vi "Microchip 93LC56BT Write.vi"() -> ()   [LabVIEW 2015]
doc: "This example shows a more generalized way to use the SPI advanced API to write data. It allows the user to change the following parameters: page size, write delay, the endianness of the address bytes, and the number of bytes in an address.\n\nThe parameters will have the following effects:\n\nTarget Page Size (bytes): This places an additional constraint on the amount of bytes written. The smaller value will be used, and that number of bytes written.\nWrite Delay Between Pages (ms): This will force a mandatory delay after writing bytes to a device.\nData Address Width: This will allow the user to specify the EEPROM Data Address as either 1 or 2 bytes.\nData Address Endianness: This control will change the ordering of the bytes in the EEPROM Data Address, note that this only has an effect if there are 2 bytes in the address.\n\nFor connection information see the NI-845x Hardware and Software manual and the manual for your specific SPI device."
uses:
  <vilib>/ni845x/ni845x.llb/ni845xControl.ctl
  <vilib>/ni845x/ni845x.llb/ni845xSpiScriptControl.ctl
  <vilib>/ni845x/ni845x.llb/NI-845x SPI Script Ms Delay.vi
  <vilib>/ni845x/ni845x.llb/NI-845x SPI Close Script Reference.vi
  <resource>/objmgr/NI845x.rc
panel:
  in  "EWEN":u8=19 format="%08b"
  in  "READ":u8=6 format="%08b"
  in  "WRITE":u8=5 format="%08b"
  in  "Read Device":bool
  in  "Program Device":bool
  out "Read Data":u16[](array[numeric]) format="%x"
  in  "EWDS":u8=16 format="%08b"
  in  "CS Idle":enum16{"Low (Assert High)", "High (Assert Low)"}(ring)
  in  "clock phase":i32(ring) items=["0 (First Edge)", "1 (Second Edge)"]
  in  "clock polarity":i32(ring) items=["0 (Idle Low)", "1 (Idle High)"]
  in  "SPI Script Reference":T1
  in  "QUIT":bool
  in  "Bit Pattern":T2(ring)
  in  "I/O Voltage Level":i32(ring)=33 items=["3.3V"=33, "2.5V"=25, "1.8V"=18, "1.5V"=15, "1.2V"=12]
  in  "Data Address Endianness":bool=TRUE
  in  "Chip Select":u32
  in  "Data Address Width":enum16{"1 Byte", "2 Byte"}(ring)
  in  "Page Write Delay (ms)":u32=3
  in  "Target Page Size (bytes)":u32=2
  in  "NI8451 Device ID":T3="NI-8451"
  in  "EEPROM Data Address":u8 format="%.0x"
  in  "Number of Bytes (Read/Write)":u32=2
  in  "Clock Rate (kHz)":u16=2000
  out "Data Bytes Written":u8[](array[numeric]) format="%x"
  # "SPI Slave Configuration"
  # "SPI Data"
  # "NI-USB-8451 Device Configuration"
  # "Big Endian"
  # "Little Endian"
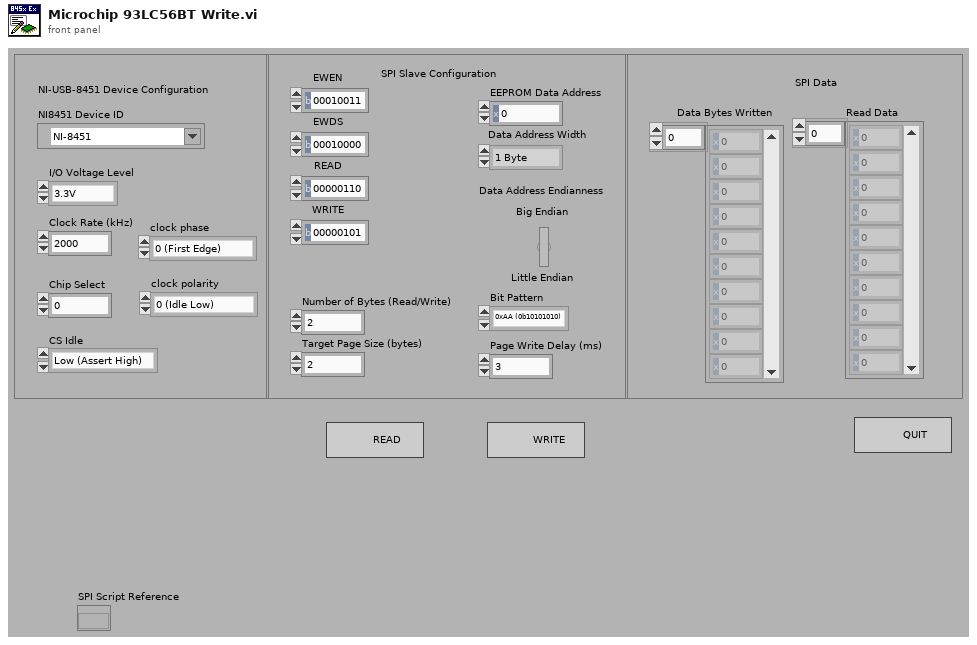
[diagram p1: front panel]
types:
  T1 = typedef "ni845xSpiScriptControl.ctl" = refnum<k20>
  T2 = enum16{"0xAA (0b10101010)", "0x55 (0b01010101)", "All ONES", "All ZEROES"}
  T3 = typedef "ni845xControl.ctl" = refnum<k21>
  T4 = enum32{"Invalid", "Standard", "Closed", "Hidden", "Minimized", "Maximized"}
  T5 = enum32{"invalid app kind", "Development System", "Run Time System", "Student Edition", "Embedded LabVIEW", "Evaluation", "Custom"}
  T6 = cluster{"SPI Script Reference":T1, "Core":cluster{"Current VI Reference":refnum<vi>, "Close Panel on Exit?":bool}, "NI8451 Device ID":T3, "I/O Voltage Level":i32, "Chip Select":u32, "Clock Rate (kHz)":u16, "clock polarity":i32, "clock phase":i32, "EEPROM Data Address":u8, "Number of Bytes (Read/Write)":u32, "Target Page Size (bytes)":u32, "Page Write Delay (ms)":u32, "CS Idle":enum16{"Low (Assert High)", "High (Assert Low)"}, "Data Address Width":enum16{"1 Byte", "2 Byte"}, "script read index":u32, "READ":u8, "WRITE":u8, "EWEN":u8, "EWDS":u8, "Data Address Endianness":bool}
  T7 = cluster{"Current VI Reference":refnum<vi>, "Close Panel on Exit?":bool}
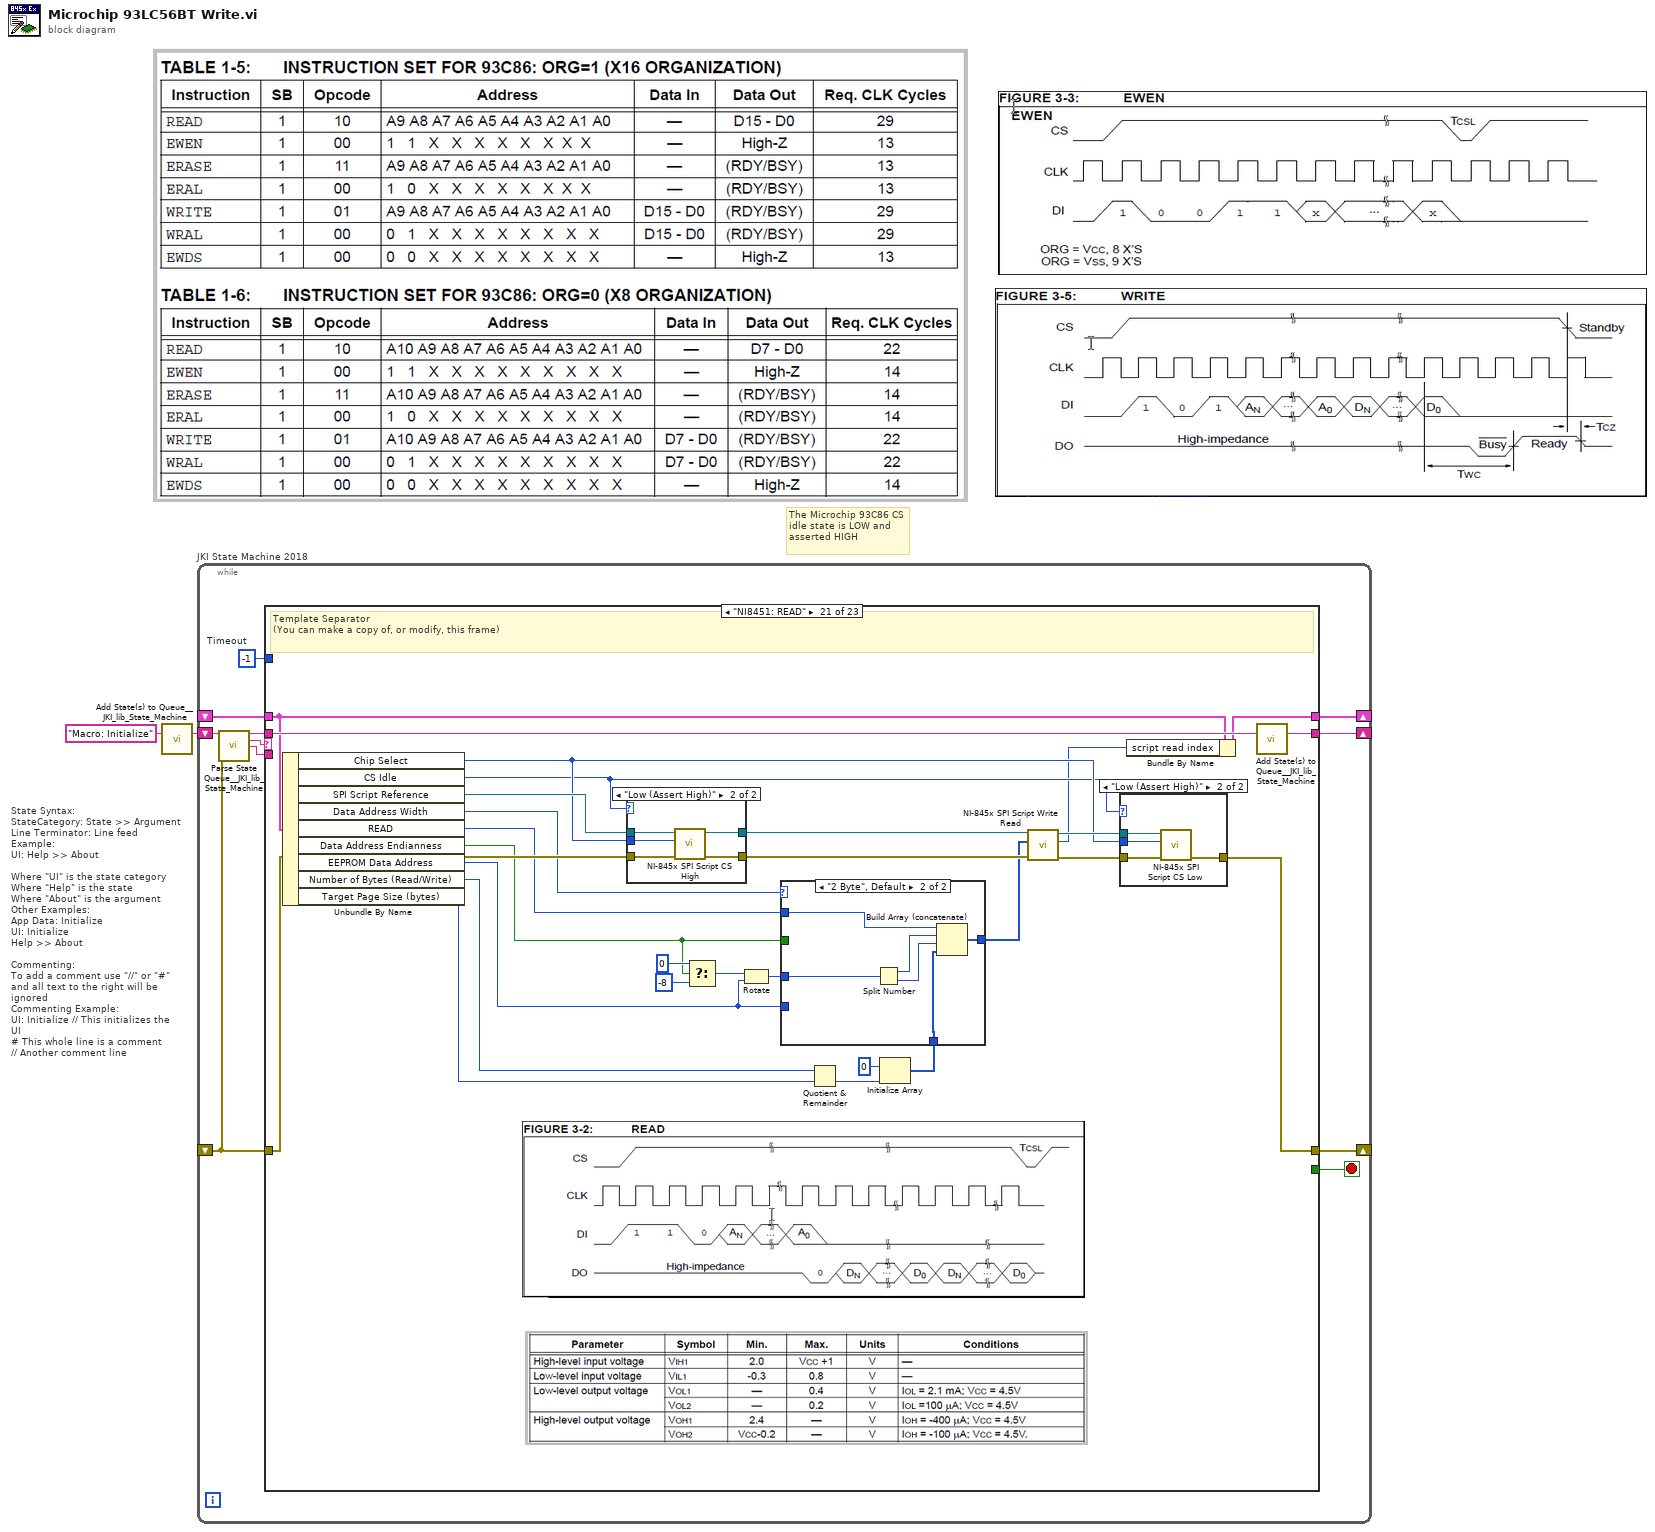
[diagram p0: block diagram]
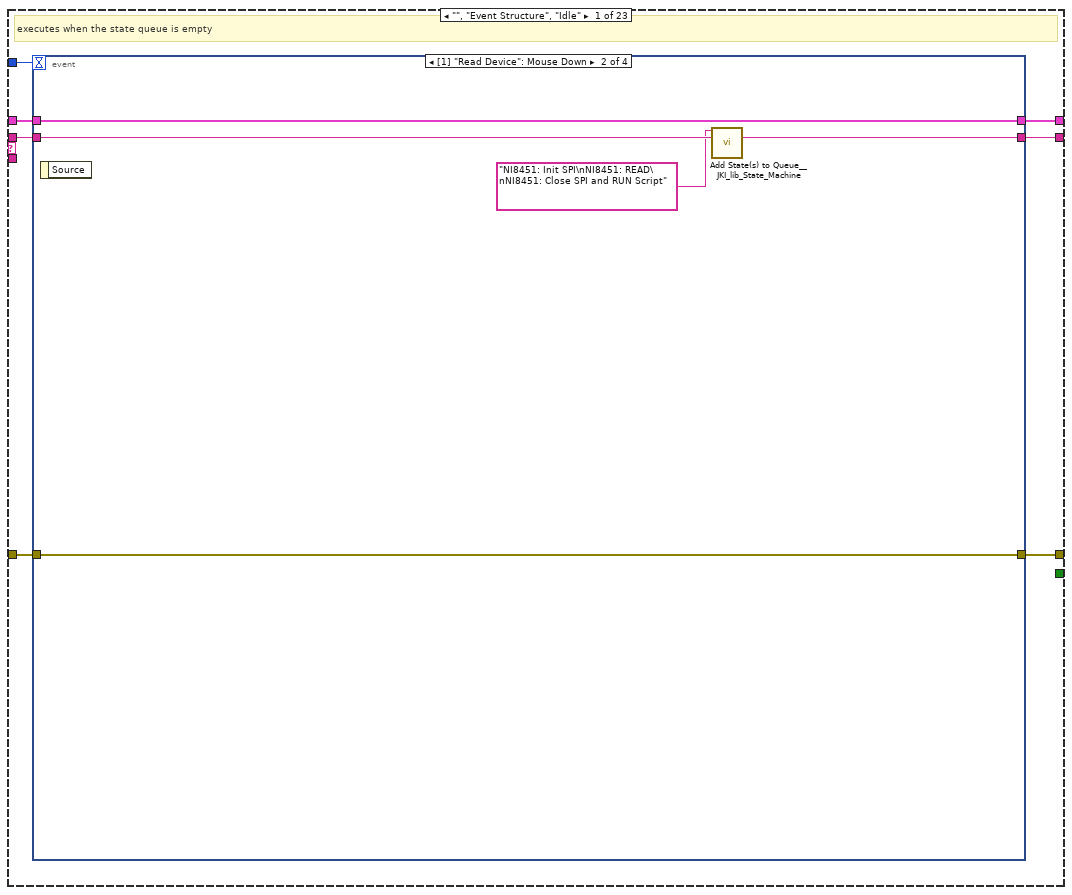
[diagram p2: hidden frame]
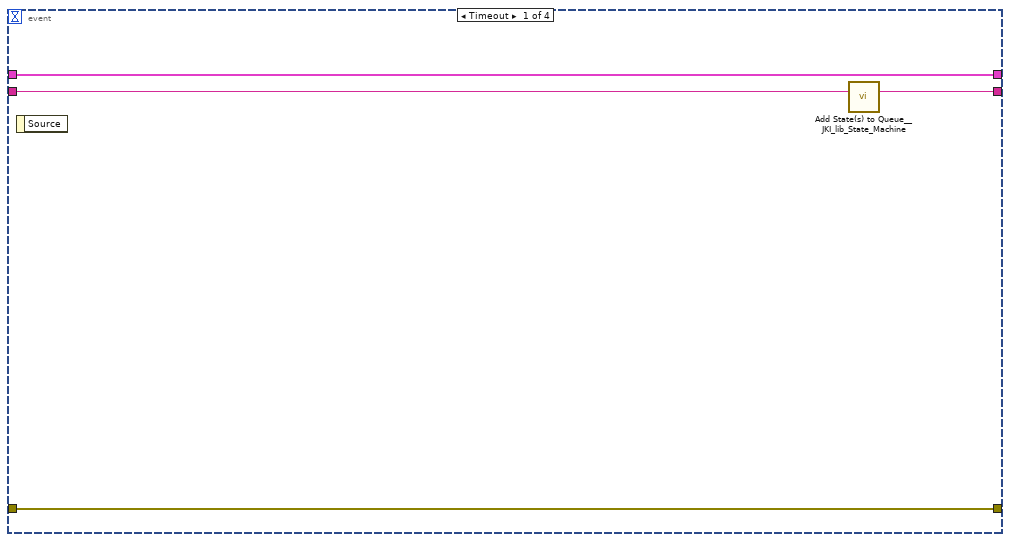
[diagram p3: hidden frame]
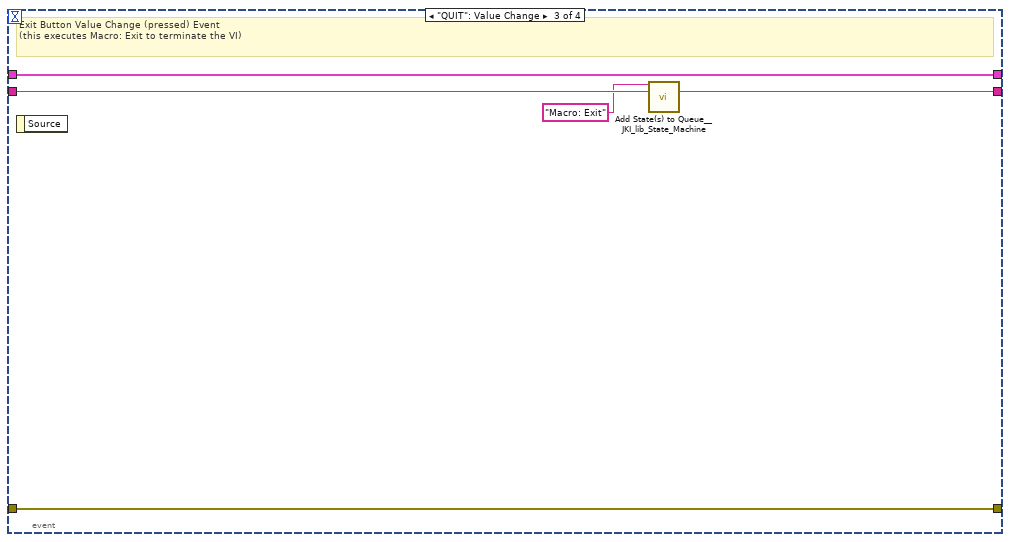
[diagram p4: hidden frame]
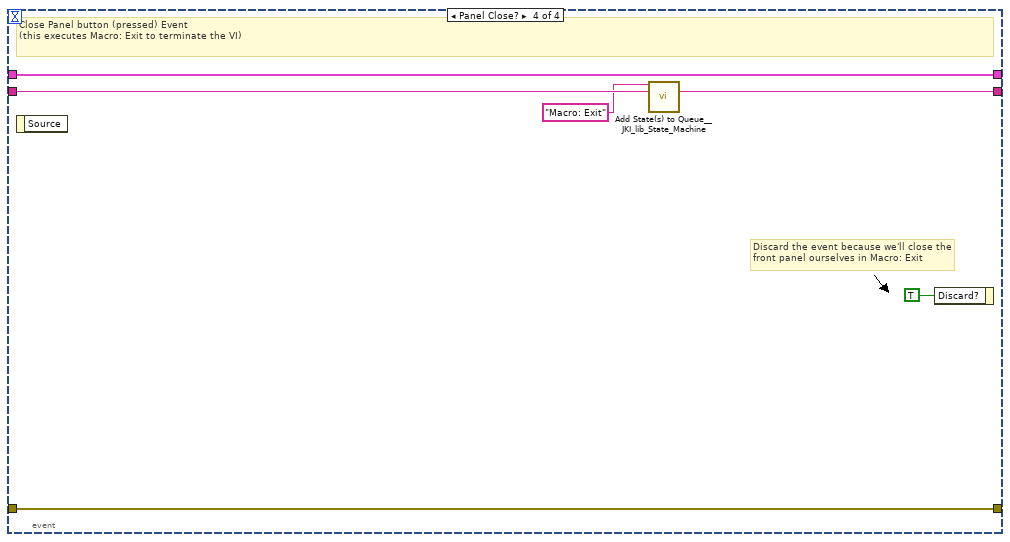
[diagram p5: hidden frame]
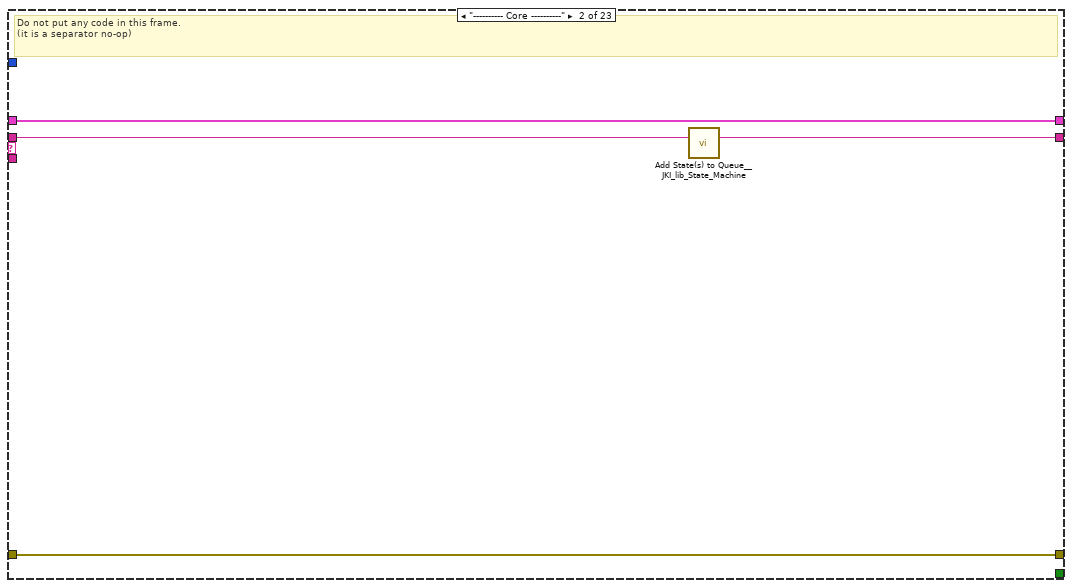
[diagram p6: hidden frame]
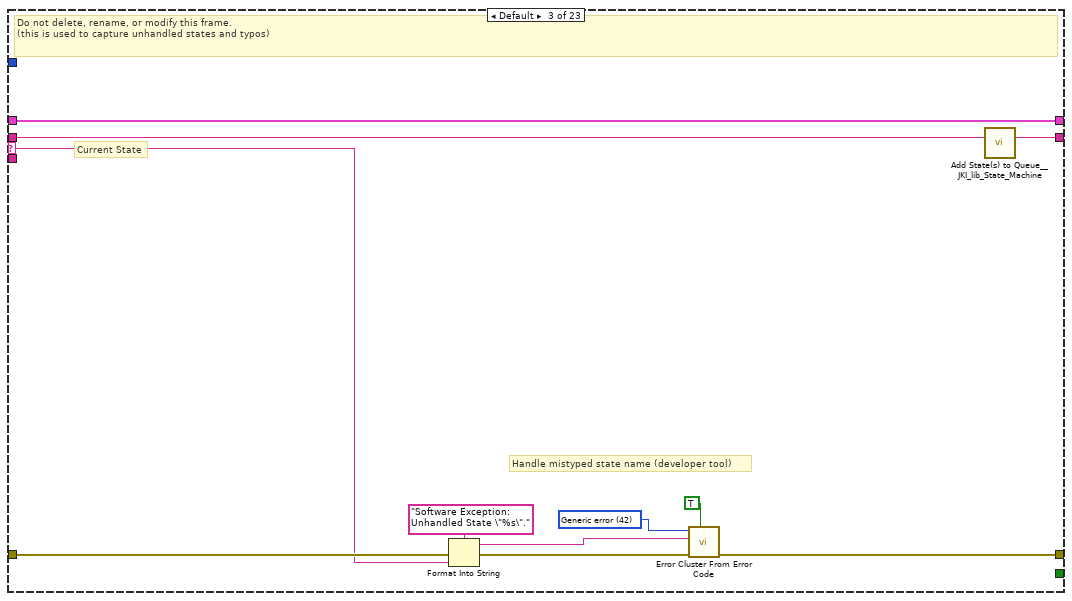
[diagram p7: hidden frame]
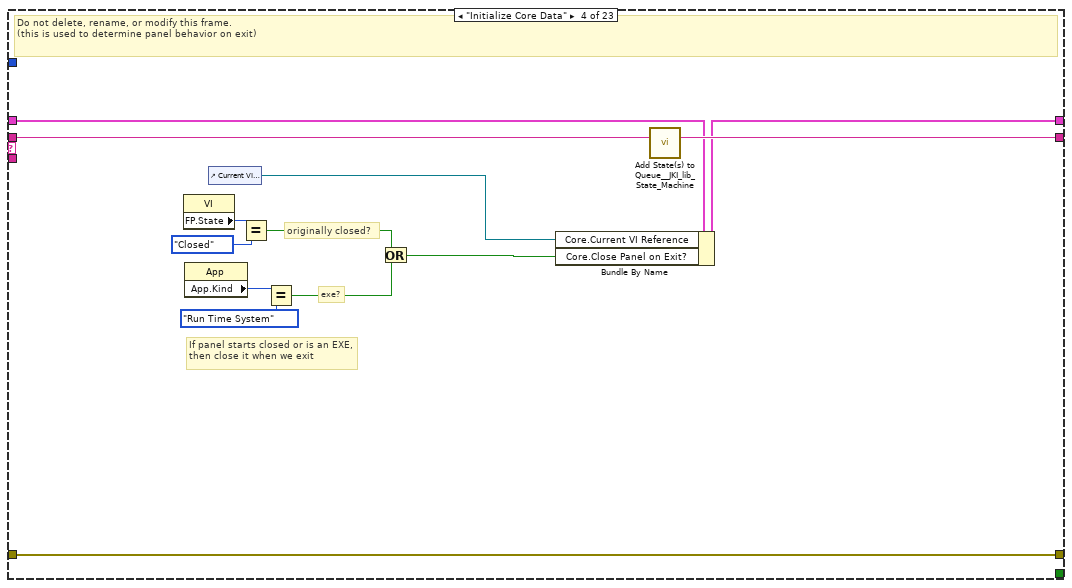
[diagram p8: hidden frame]
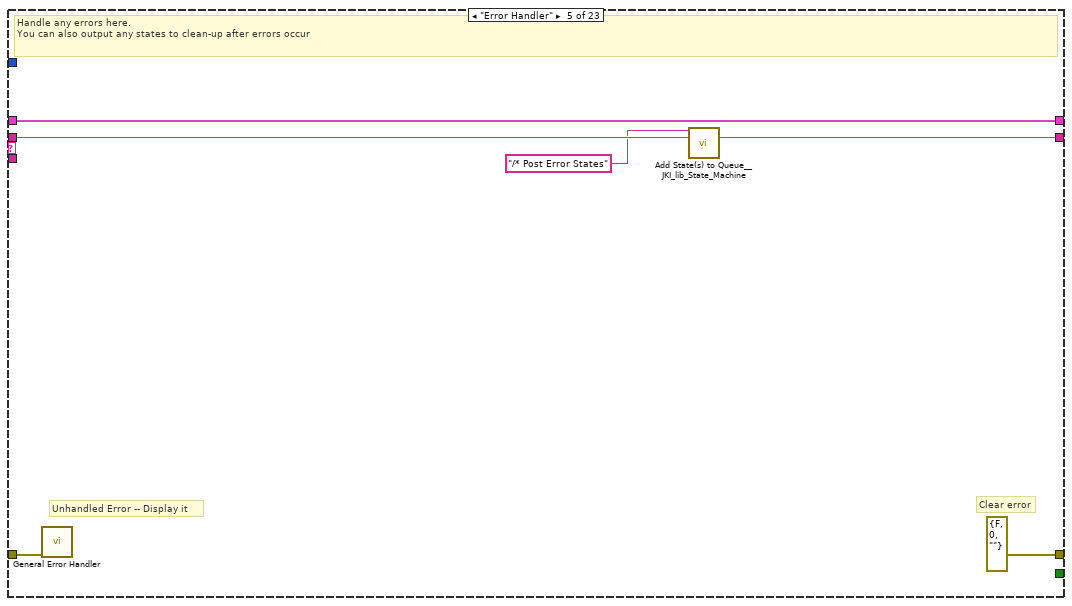
[diagram p9: hidden frame]
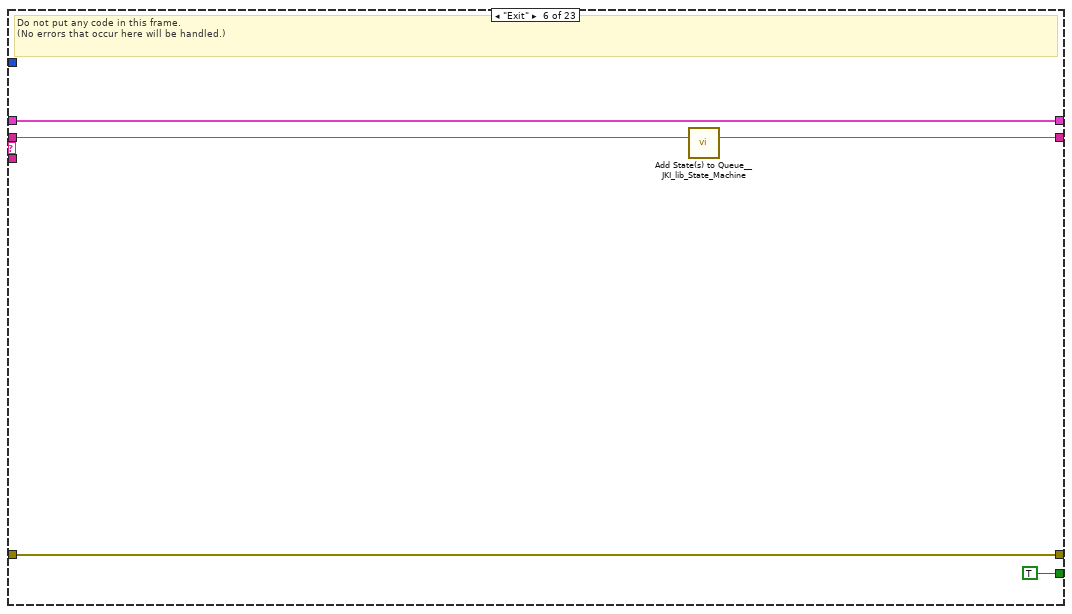
[diagram p10: hidden frame]
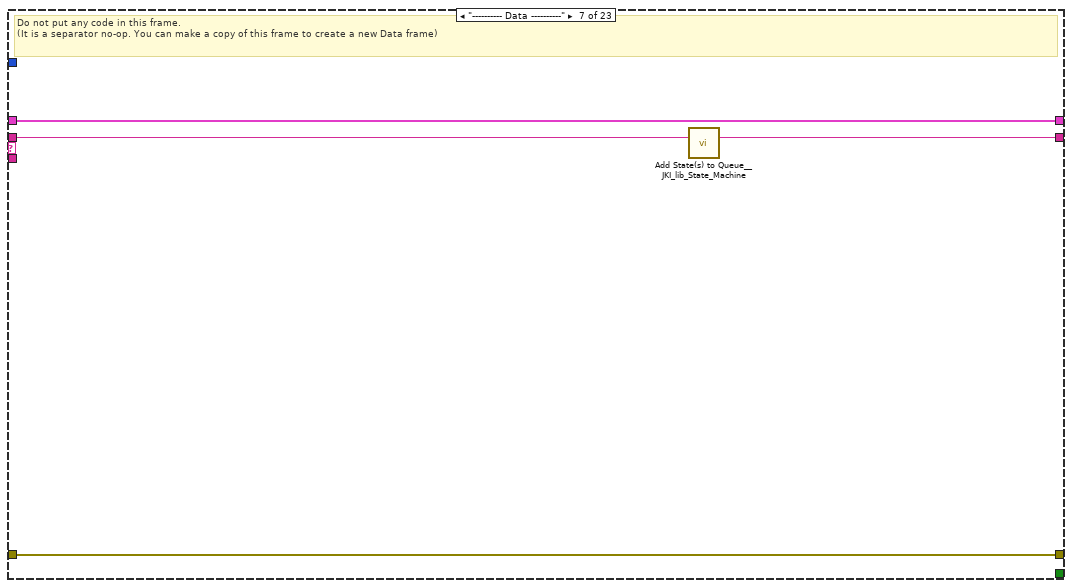
[diagram p11: hidden frame]
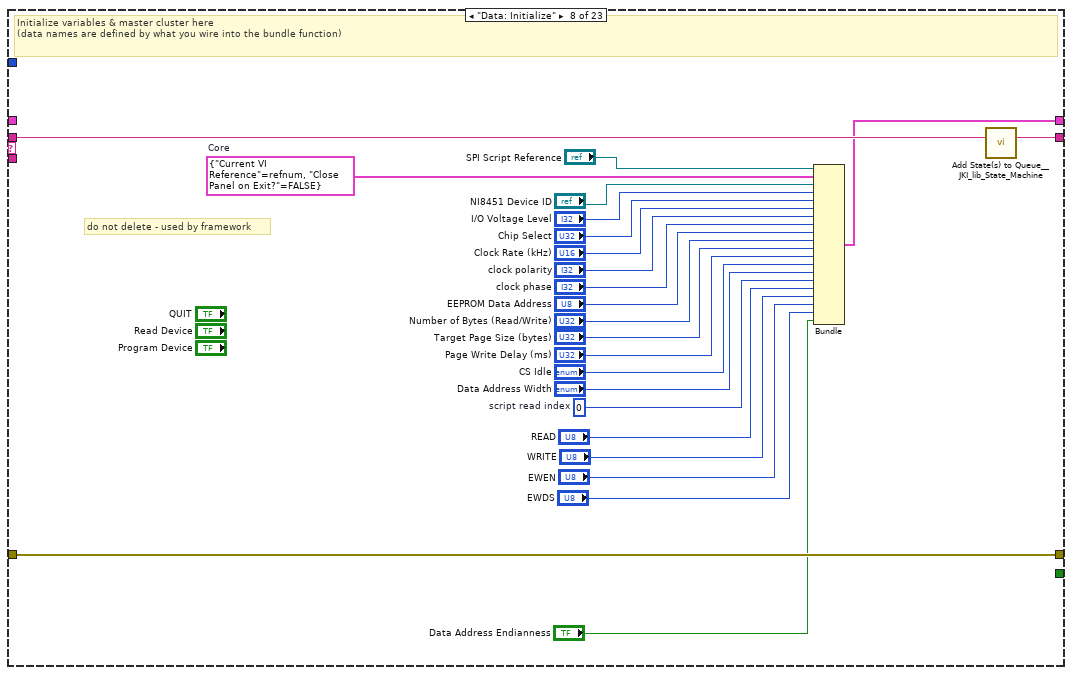
[diagram p12: hidden frame]
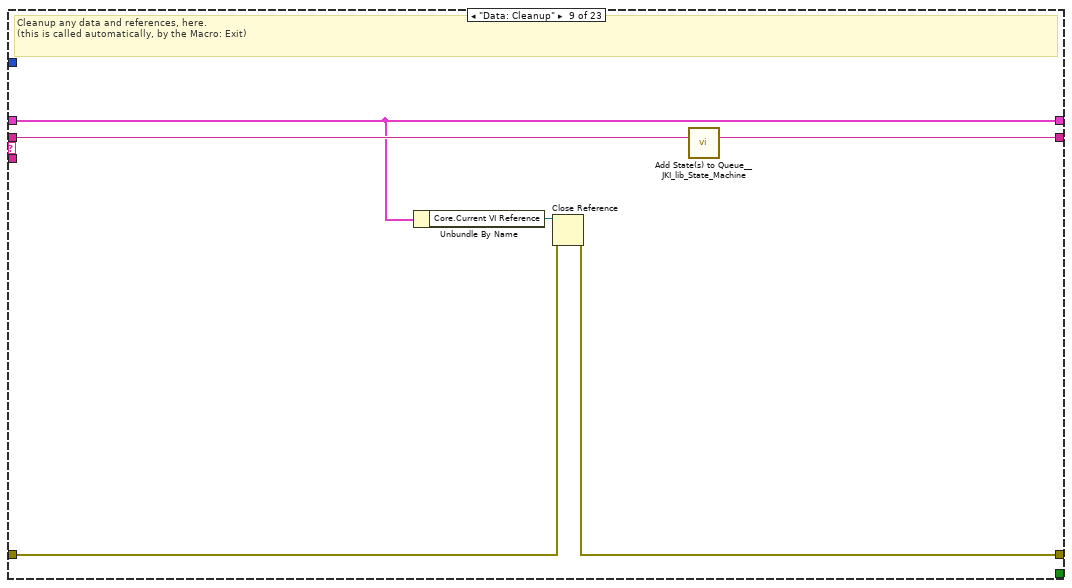
[diagram p13: hidden frame]
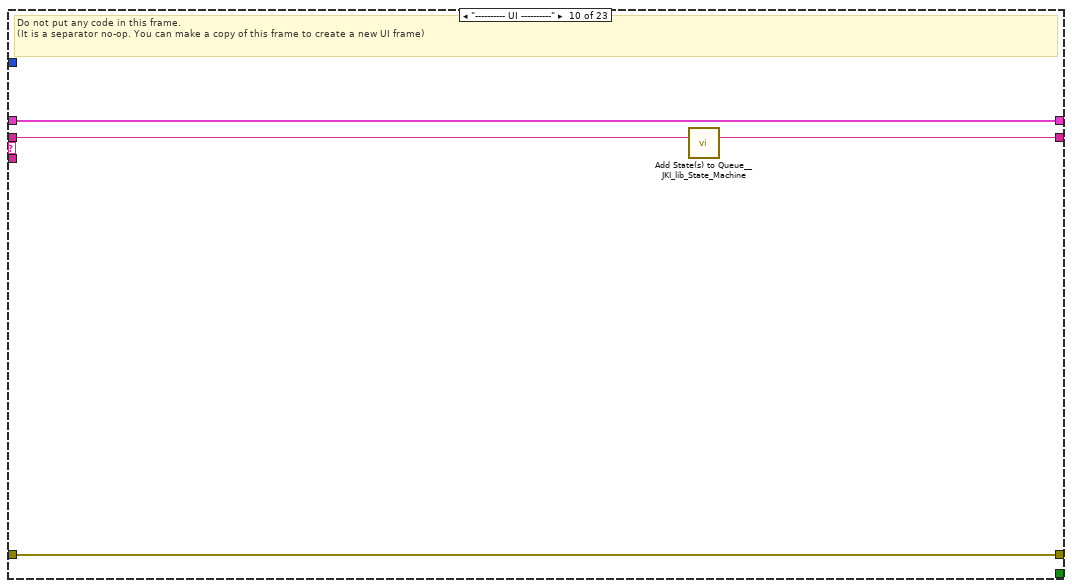
[diagram p14: hidden frame]
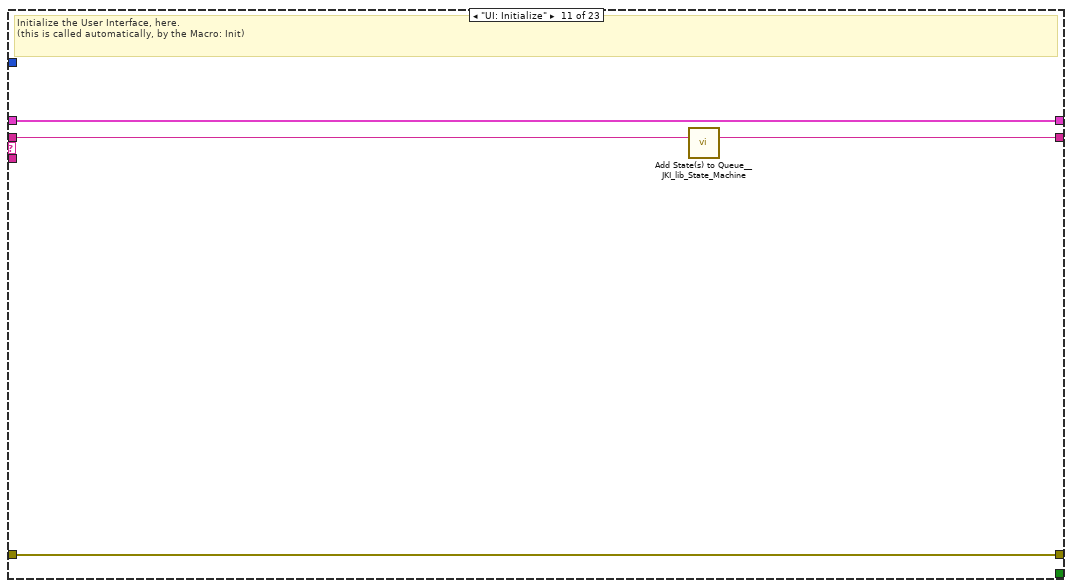
[diagram p15: hidden frame]
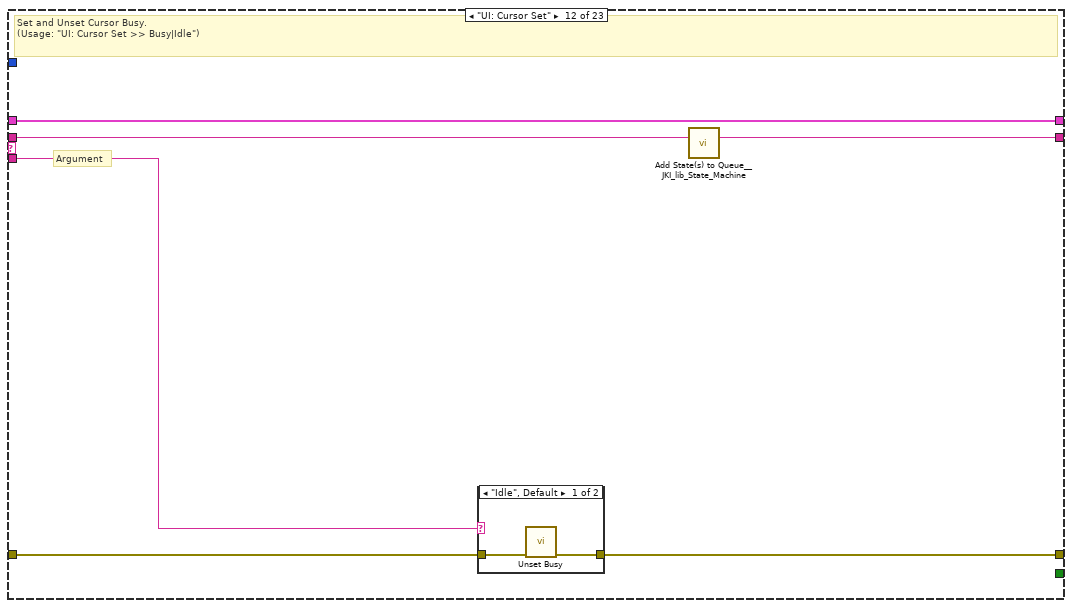
[diagram p16: hidden frame]
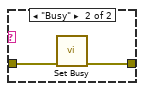
[diagram p17: hidden frame]
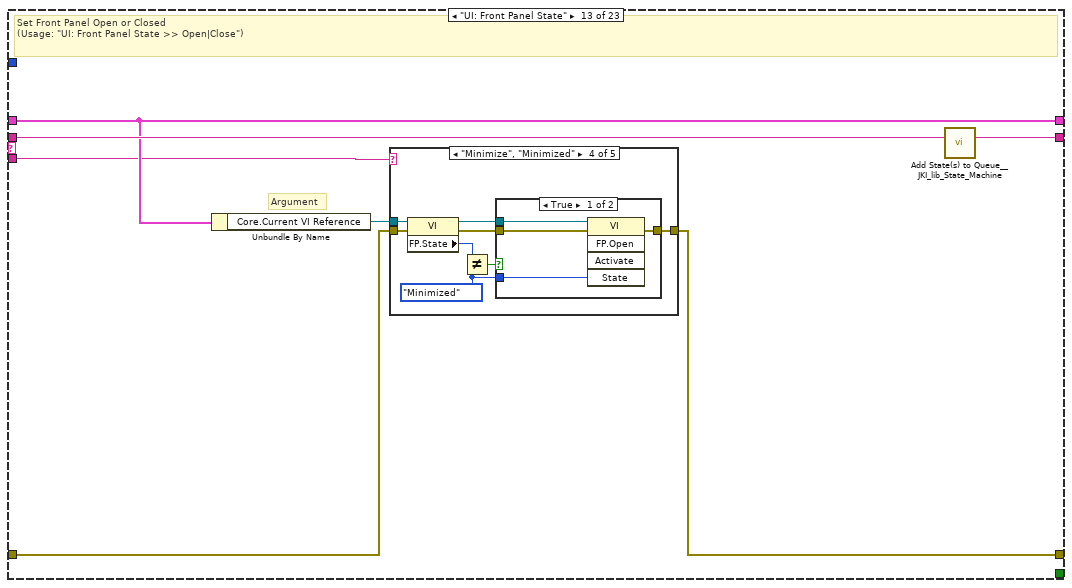
[diagram p18: hidden frame]
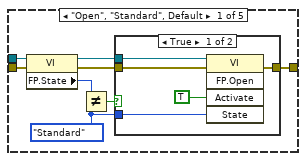
[diagram p19: hidden frame]
diagram:
  # "The Microchip 93C86 CS idle state is LOW and asserted HIGH"
  # "State Syntax:\nStateCategory: State >> Argument\nLine Terminator: Line feed\nExample:\nUI: Help >> About\n\nWhere \"UI\" is the state category\nWhere \"Help\" is the state\nWhere \"About\" is the argument\nOther Examples:\nApp Data: Initialize\nUI: Initialize\nHelp >> About\n\nCommenting:\nTo add a comment use \"//\" or \"#\" and all text to the right will be ignored\nCommenting Example:\nUI: Initialize // This initializes the UI\n# This whole line is a comment\n// Another comment line"
  n1 = call <vilib>:"Add State(s) to Queue__JKI_lib_State_Machine.vi"("State(s) in (\"\")"="Macro: Initialize") -> ("States Out"=w2:string)  [unwired: 14 in]
  n2 = while "JKI State Machine 2018" {
    shift-right: [w6] -> _
    shift-left: _ -> [w5]
    shift-right: [w9] -> _
    shift-left: _ -> [w3]
    shift-right: [w8] -> _
    shift-left: w2 -> [w10]
    stop <- w7 stop-if-true
    w4 = -1  # Timeout
    n3 = call <vilib>:"Parse State Queue__JKI_lib_State_Machine.vi"("State Queue"=w10, "Error In (no error)"=w3) -> ("Remaining States"=w12:string, "Current State"=w13:string, "Arguments"=w11:string)  [unwired: 11 in]
    n4 = case shown="\"NI8451: READ\"" w13 {
      selector: w13 -> [_ _ w45 _ _ _ _ _ _ _ _ _ _ _ _ _ _ _ _ _ _ _ _]
      tunnel: w12 -> [w20 w44 w49 w68 w74 w79 w83 w107 w113 w117 w121 w127 w138 w207 w212 w222 w226 w248 w270 w304 w402 w456 w474]
      tunnel: w11 -> [_ _ _ _ _ _ _ _ _ _ _ w122 w132 _ _ _ _ _ _ _ _ _ _]
      tunnel: w5 -> [w18 w41 w47 w61 w71 w77 w80 _ w108 w114 w119 w125 w134 w204 w209 w219 w223 w238 w260 w296 w386 w448 w467]
      tunnel: [w17 w42 w51 w65 errorcluster {"status"=FALSE, "code"=0, "source"=""} ("error out") w76 w81 w104 w109 w115 w118 w123 w135 w205 w210 w220 w224 w230 w261 w297 w384 w449 w469] -> w9
      tunnel: w3 -> [w16 w42 w50 w65 w70 w76 w81 w104 w110 w115 w118 w124 w136 w205 w210 w220 w224 w231 w262 w298 w385 w450 w470]
      tunnel: [w19 w43 w48 w67 w73 w78 w82 w106 w112 w116 w120 w126 w137 w206 w211 w221 w225 w247 w269 w303 w401 w455 w473] -> w8
      tunnel: [_ _ _ _ _ TRUE _ _ _ _ _ _ _ _ _ _ _ _ _ _ _ _ _] -> w7
      tunnel: [w15 w41 w47 w66 w71 w77 w80 w105 w108 w114 w119 w125 w134 w204 w209 w219 w223 w235 w260 w288 w376 w448 w467] -> w6
      tunnel: w4 -> [w14 _ _ _ _ _ _ _ _ _ _ _ _ _ _ _ _ _ _ _ _ _ _]
      frame "", "Event Structure", "Idle" {
        # "executes when the state queue is empty"
        n5 = event shown="[1] \"Read Device\": Mouse Down" {
          selector: _ -> [_ _ _ _]
          dyn-events: _ -> [_ _ _ _]
          timeout: w14 -> [_ _ _ _]
          tunnel: w20 -> [w24 w27 w34 w40]
          tunnel: [w23 w26 w33 w39] -> w19
          tunnel: w18 -> [w21 w29 w31 w37]
          tunnel: [w22 w28 w32 w38] -> w17
          tunnel: w16 -> [w22 w28 w32 w38]
          tunnel: [w21 w29 w31 w37] -> w15
          event Timeout {
            n6 = event-data() -> ()  [unwired: 1 in, 1 out]
            n7 = call <vilib>:"Add State(s) to Queue__JKI_lib_State_Machine.vi"("State(s) in (\"\")"=w24) -> ("States Out"=w23:string)  [unwired: 14 in]
          }
          event "Read Device": Mouse Down {
            n8 = event-data() -> ()  [unwired: 1 in, 1 out]
            n9 = call <vilib>:"Add State(s) to Queue__JKI_lib_State_Machine.vi"("State(s) in Front (\"\")"="NI8451: Init SPI\nNI8451: READ\nNI8451: Close SPI and RUN Script" ("State(s) in Front (\"\")"), "State(s) in (\"\")"=w27) -> ("States Out"=w26:string)  [unwired: 13 in]
          }
          event "QUIT": Value Change {
            # "Exit Button Value Change (pressed) Event\n(this executes Macro: Exit to terminate the VI)"
            n10 = event-data() -> ()  [unwired: 1 in, 1 out]
            n11 = call <vilib>:"Add State(s) to Queue__JKI_lib_State_Machine.vi"("State(s) in Front (\"\")"="Macro: Exit", "State(s) in (\"\")"=w34) -> ("States Out"=w33:string)  [unwired: 13 in]
          }
          event Panel Close? {
            # "Discard the event because we'll close the front panel ourselves in Macro: Exit"
            # "Close Panel button (pressed) Event\n(this executes Macro: Exit to terminate the VI)"
            n12 = event-data() -> ()  [unwired: 1 in, 1 out]
            n13 = call <vilib>:"Add State(s) to Queue__JKI_lib_State_Machine.vi"("State(s) in Front (\"\")"="Macro: Exit", "State(s) in (\"\")"=w40) -> ("States Out"=w39:string)  [unwired: 13 in]
            n14 = event-data("Discard?"=TRUE) -> ()  [unwired: 1 in, 1 out]
          }
        }
      }
      frame "---------- Core ----------" {
        # "Do not put any code in this frame.\n(it is a separator no-op)"
        n15 = call <vilib>:"Add State(s) to Queue__JKI_lib_State_Machine.vi"("State(s) in (\"\")"=w44) -> ("States Out"=w43:string)  [unwired: 14 in]
      }
      frame Default {
        w54 = 42 items=["No error", "Argument error", "Memory is full", "Out of zone", "End of file", "File already open", "Generic file I/O error", "File not found", "File permission error", "Disk is full", "Duplicate path", "Too many files open", "System feature not enabled", "Resource file not found", "Cannot add resource", "Resource not found", "Image not found", "Image memory error", "Pen does not exist", "Config type invalid", "Config token not found", "Config parse error", "Config memory error", "Bad external code format", "Bad external code offset", "External code not present", "Null window", "Destroy window error", "Null menu", "Print aborted", "Bad print record", "Print driver error", "Windows error during printing", "Memory error during printing", "Print dialog error", "Generic print error", "Invalid device refnum", "Device not found", "Device parameter error", "Device unit error", "Cannot open device", "Device call aborted", "Generic error", "Cancelled by user", "Object ID too low", "Object ID too high", "Object not in heap", "Unknown heap", "Unknown object (invalid DefProc)", "Unknown object (DefProc not in table)", "Message out of range", "Invalid (null) method", "Unknown message", "Manager call not supported", "Bad address", "Network operation in progress", "Network operation timed out", "Connection is busy", "Network attribute not supported", "Network error", "Address in use", "System out of memory", "Connection aborted", "Connection refused", "Not connected", "Already connected", "Connection closed", "Initialization error (interapplication manager)", "Bad occurrence", "Wait on unbound occurrence handler", "Occurrence queue overflow", "Datalog type conflict", "Unused", "Unrecognized type (interapplication manager)", "Memory corrupt", "Failed to make temporary DLL", "Old CIN version", "Drag socket not found", "Failed to load drop-object", "Failed to register OLE object", "Failed to release OLE object", "Format specifier type mismatch", "Unknown format specifier", "Too few format specifiers", "Too many format specifiers", "Scan failed", "Newer CIN version", "Error converting to variant", "Runtime menu error", "Password tampered", "Variant attribute not found", "Incompatible variant data type", "Event data is not available", "Event Store is not present", "Occurrence is not found", "Event Queue is not created", "Event info is not available", "Refnum passed is NULL", "Error retrieving Class GUID", "Error retrieving CoClass GUID", "Error retrieving TypeLib GUID.", "Bad built application magic bytes.", "Specific driver is different from the specific driver associated with the Logical Name.", "There is no session opened to the class driver.", "Max Error", "MAX - Error with config objects", "MAX - Error loading configuration", "MAX - Group not supported"]
        # "Current State"
        # "Handle mistyped state name (developer tool)"
        # "Do not delete, rename, or modify this frame.\n(this is used to capture unhandled states and typos)"
        n16 = Format Into String(format string="Software Exception: Unhandled State \"%s\"." ("message"), error in=w50, w45) -> (resulting string=w53:string, error out=w52:errorcluster)  [unwired: 1 in]
        n17 = call <vilib>:"Error Cluster From Error Code.vi"("show call chain? (False)"=TRUE, "error in (no error)"=w52, "error message (\"\")"=w53, "error code (0)"=w54) -> ("error out"=w51:errorcluster)  [unwired: 5 in]
        n18 = call <vilib>:"Add State(s) to Queue__JKI_lib_State_Machine.vi"("State(s) in (\"\")"=w49) -> ("States Out"=w48:string)  [unwired: 14 in]
      }
      frame "Initialize Core Data" {
        # "originally closed?"
        # "exe?"
        # "If panel starts closed or is an EXE, then close it when we exit"
        # "Do not delete, rename, or modify this frame.\n(this is used to determine panel behavior on exit)"
        n19 = property class="VI"() -> ("FP.State"=w58:T4)  [unwired: 2 in, 2 out]
        n20 = property class="App"() -> ("App.Kind"=w64:T5)  [unwired: 2 in, 2 out]
        n21 = control-ref of="Current VI Reference"() -> (w59:refnum<vi>)
        n22 = Equal?(x=w58, y=T4."Closed" ("Front Panel Window:State")) -> (x = y?=w56:bool)
        n23 = Equal?(x=w64, y=T5."Run Time System" ("Application:Kind")) -> (x = y?=w62:bool)
        n24 = Or(x=w56, y=w62) -> (x .or. y?=w60:bool)
        n25 = Bundle By Name(cluster=w61, "Core.Current VI Reference"=w59, "Core.Close Panel on Exit?"=w60) -> (w66:T6)
        n26 = call <vilib>:"Add State(s) to Queue__JKI_lib_State_Machine.vi"("State(s) in (\"\")"=w68) -> ("States Out"=w67:string)  [unwired: 14 in]
      }
      frame "Error Handler" {
        # "Unhandled Error -- Display it"
        # "Clear error"
        # "Handle any errors here.\nYou can also output any states to clean-up after errors occur"
        n27 = call <vilib>:"General Error Handler.vi"("error in (no error)"=w70) -> ()  [unwired: 10 in, 5 out]
        n28 = call <vilib>:"Add State(s) to Queue__JKI_lib_State_Machine.vi"("State(s) in Front (\"\")"="/* Post Error States", "State(s) in (\"\")"=w74) -> ("States Out"=w73:string)  [unwired: 13 in]
      }
      frame "Exit" {
        # "Do not put any code in this frame.\n(No errors that occur here will be handled.)"
        n29 = call <vilib>:"Add State(s) to Queue__JKI_lib_State_Machine.vi"("State(s) in (\"\")"=w79) -> ("States Out"=w78:string)  [unwired: 14 in]
      }
      frame "---------- Data ----------" {
        # "Do not put any code in this frame.\n(It is a separator no-op. You can make a copy of this frame to create a new Data frame)"
        n30 = call <vilib>:"Add State(s) to Queue__JKI_lib_State_Machine.vi"("State(s) in (\"\")"=w83) -> ("States Out"=w82:string)  [unwired: 14 in]
      }
      frame "Data: Initialize" {
        w88 = u32 0  # script read index
        w103 = T7 {"Current VI Reference"=refnum, "Close Panel on Exit?"=FALSE}  # Core
        # "do not delete - used by framework"
        # "Initialize variables & master cluster here\n(data names are defined by what you wire into the bundle function)"
        n31 = Bundle("SPI Script Reference"="SPI Script Reference", "Core"=w103, "NI8451 Device ID"="NI8451 Device ID", "I/O Voltage Level"="I/O Voltage Level", "Chip Select"="Chip Select", "Clock Rate (kHz)"="Clock Rate (kHz)", "clock polarity"="clock polarity", "clock phase"="clock phase", "EEPROM Data Address"="EEPROM Data Address", "Number of Bytes (Read/Write)"="Number of Bytes (Read/Write)", "Target Page Size (bytes)"="Target Page Size (bytes)", "Page Write Delay (ms)"="Page Write Delay (ms)", "CS Idle"="CS Idle", "Data Address Width"="Data Address Width", "script read index"=w88, "READ"="READ", "WRITE"="WRITE", "EWEN"="EWEN", "EWDS"="EWDS", "Data Address Endianness"="Data Address Endianness") -> (w105:T6)  [unwired: 1 in]
        n32 = call <vilib>:"Add State(s) to Queue__JKI_lib_State_Machine.vi"("State(s) in (\"\")"=w107) -> ("States Out"=w106:string)  [unwired: 14 in]
      }
      frame "Data: Cleanup" {
        # "Cleanup any data and references, here.\n(this is called automatically, by the Macro: Exit)"
        n33 = Unbundle By Name(w108) -> ("Core.Current VI Reference"=w111:refnum<vi>)
        n34 = Close Reference(reference=w111, error in (no error)=w110) -> (error out=w109:errorcluster)
        n35 = call <vilib>:"Add State(s) to Queue__JKI_lib_State_Machine.vi"("State(s) in (\"\")"=w113) -> ("States Out"=w112:string)  [unwired: 14 in]
      }
      frame "---------- UI ----------" {
        # "Do not put any code in this frame.\n(It is a separator no-op. You can make a copy of this frame to create a new UI frame)"
        n36 = call <vilib>:"Add State(s) to Queue__JKI_lib_State_Machine.vi"("State(s) in (\"\")"=w117) -> ("States Out"=w116:string)  [unwired: 14 in]
      }
      frame "UI: Initialize" {
        # "Initialize the User Interface, here.\n(this is called automatically, by the Macro: Init)"
        n37 = call <vilib>:"Add State(s) to Queue__JKI_lib_State_Machine.vi"("State(s) in (\"\")"=w121) -> ("States Out"=w120:string)  [unwired: 14 in]
      }
      frame "UI: Cursor Set" {
        # "Argument"
        # "Set and Unset Cursor Busy.\n(Usage: \"UI: Cursor Set >> Busy|Idle\")"
        n38 = case shown="\"Idle\", Default" w122 {
          tunnel: w124 -> [w129 w131]
          tunnel: [w128 w130] -> w123
          frame "Idle", Default {
            n39 = call <vilib>:"Unset Busy.vi"("error in (no error)"=w129) -> ("error out"=w128:errorcluster)  [unwired: 10 in]
          }
          frame "Busy" {
            n40 = call <vilib>:"Set Busy.vi"("error in (no error)"=w131) -> ("error out"=w130:errorcluster)  [unwired: 9 in, 1 out]
          }
        }
        n41 = call <vilib>:"Add State(s) to Queue__JKI_lib_State_Machine.vi"("State(s) in (\"\")"=w127) -> ("States Out"=w126:string)  [unwired: 14 in]
      }
      frame "UI: Front Panel State" {
        # "Argument"
        # "Set Front Panel Open or Closed\n(Usage: \"UI: Front Panel State >> Open|Close\")"
        n42 = Unbundle By Name(w134) -> ("Core.Current VI Reference"=w133:refnum<vi>)
        n43 = case shown="\"Minimize\", \"Minimized\"" w132 {
          tunnel: w136 -> [w144 w159 w170 w183 w196]
          tunnel: [w146 w160 w172 w185 w198] -> w135
          tunnel: w133 -> [w145 w157 w171 w184 w197]
          frame "Open", "Standard", Default {
            w139 = T4."Standard" ("State")
            n44 = property class="VI"(reference=w145, error in=w144) -> (reference out=w142:refnum<vi>, error out=w143:errorcluster, "FP.State"=w141:T4)
            n45 = Not Equal?(x=w141, y=w139) -> (x != y?=w140:bool)
            n46 = case shown="True" w140 {
              tunnel: [w150 w152] -> w146
              tunnel: w143 -> [w149 w152]
              tunnel: w142 -> [w148 _]
              tunnel: w139 -> [w147 _]
              frame True {
                n47 = invoke class="VI" method="FP.Open"(reference=w148, error in=w149, "Activate"=TRUE, "State"=w147) -> (error out=w150:errorcluster)  [unwired: 1 in, 4 out]
              }
              frame False {
              }
            }
          }
          frame "Close", "Closed" {
            n48 = property class="VI"(reference=w157, error in=w159) -> (reference out=w156:refnum<vi>, error out=w158:errorcluster, "FP.State"=w154:T4)
            n49 = Not Equal?(x=w154, y=T4."Closed" ("Front Panel Window:State")) -> (x != y?=w153:bool)
            n50 = case shown="True" w153 {
              tunnel: [w161 w164] -> w160
              tunnel: w158 -> [w161 w163]
              tunnel: w156 -> [_ w162]
              frame False {
              }
              frame True {
                n51 = invoke class="VI" method="FP.Close"(reference=w162, error in=w163) -> (error out=w164:errorcluster)  [unwired: 1 in, 2 out]
              }
            }
          }
          frame "Hidden", "Hide" {
            w165 = T4."Hidden" ("State")
            n52 = property class="VI"(reference=w171, error in=w170) -> (reference out=w168:refnum<vi>, error out=w169:errorcluster, "FP.State"=w167:T4)
            n53 = Not Equal?(x=w167, y=w165) -> (x != y?=w166:bool)
            n54 = case shown="True" w166 {
              tunnel: [w176 w177] -> w172
              tunnel: w169 -> [w175 w177]
              tunnel: w168 -> [w174 _]
              tunnel: w165 -> [w173 _]
              frame True {
                n55 = invoke class="VI" method="FP.Open"(reference=w174, error in=w175, "State"=w173) -> (error out=w176:errorcluster)  [unwired: 2 in, 4 out]
              }
              frame False {
              }
            }
          }
          frame "Minimize", "Minimized" {
            w178 = T4."Minimized" ("State")
            n56 = property class="VI"(reference=w184, error in=w183) -> (reference out=w181:refnum<vi>, error out=w182:errorcluster, "FP.State"=w180:T4)
            n57 = Not Equal?(x=w180, y=w178) -> (x != y?=w179:bool)
            n58 = case shown="True" w179 {
              tunnel: [w189 w190] -> w185
              tunnel: w182 -> [w188 w190]
              tunnel: w181 -> [w187 _]
              tunnel: w178 -> [w186 _]
              frame True {
                n59 = invoke class="VI" method="FP.Open"(reference=w187, error in=w188, "State"=w186) -> (error out=w189:errorcluster)  [unwired: 2 in, 4 out]
              }
              frame False {
              }
            }
          }
          frame "Maximize", "Maximized" {
            w191 = T4."Maximized" ("State")
            n60 = property class="VI"(reference=w197, error in=w196) -> (reference out=w194:refnum<vi>, error out=w195:errorcluster, "FP.State"=w193:T4)
            n61 = Not Equal?(x=w193, y=w191) -> (x != y?=w192:bool)
            n62 = case shown="True" w192 {
              tunnel: [w202 w203] -> w198
              tunnel: w195 -> [w201 w203]
              tunnel: w194 -> [w200 _]
              tunnel: w191 -> [w199 _]
              frame True {
                n63 = invoke class="VI" method="FP.Open"(reference=w200, error in=w201, "State"=w199) -> (error out=w202:errorcluster)  [unwired: 2 in, 4 out]
              }
              frame False {
              }
            }
          }
        }
        n64 = call <vilib>:"Add State(s) to Queue__JKI_lib_State_Machine.vi"("State(s) in (\"\")"=w138) -> ("States Out"=w137:string)  [unwired: 14 in]
      }
      frame "---------- Macro ----------" {
        # "Do not put any code in this frame.\n(It is a separator no-op. You can make a copy of this frame to create a new Macro frame)"
        n65 = call <vilib>:"Add State(s) to Queue__JKI_lib_State_Machine.vi"("State(s) in (\"\")"=w207) -> ("States Out"=w206:string)  [unwired: 14 in]
      }
      frame "Macro: Initialize" {
        w208 = "Data: Initialize\nInitialize Core Data\nUI: Initialize\nUI: Front Panel State >> Open"  # Data: Initialize Initialize Core Data UI: Initialize UI: Front Panel State >> Open
        # "Initialization Macro\n(This is called once, when the VI starts)"
        n66 = call <vilib>:"Add State(s) to Queue__JKI_lib_State_Machine.vi"("State(s) in Front (\"\")"=w208, "State(s) in (\"\")"=w212) -> ("States Out"=w211:string)  [unwired: 13 in]
      }
      frame "Macro: Exit" {
        # "Exit Macro\n(This is called once, when the VI exits)"
        n67 = Unbundle By Name(w219) -> ("Core.Close Panel on Exit?"=w218:bool)
        n68 = Select(t="UI: Front Panel State >> Close", s=w218, f="") -> (s? t:f=w215:string)
        n69 = call <vilib>:"Add State(s) to Queue__JKI_lib_State_Machine.vi"("State(s) in (\"\")"=w215, "State(s) at Back (\"\")"="Data: Cleanup\nExit") -> ("States Out"=w213:string)  [unwired: 13 in]
        n70 = call <vilib>:"Add State(s) to Queue__JKI_lib_State_Machine.vi"("State(s) in Front (\"\")"=w213, "State(s) in (\"\")"=w222) -> ("States Out"=w221:string)  [unwired: 13 in]
      }
      frame "---------- New Category ----------" {
        # "Template Separator\n(You can make a copy of, or modify, this frame)"
        n71 = call <vilib>:"Add State(s) to Queue__JKI_lib_State_Machine.vi"("State(s) in (\"\")"=w226) -> ("States Out"=w225:string)  [unwired: 14 in]
      }
      frame "NI8451: Init SPI" {
        # "Step 1: Set the I/O reference voltage. Not all NI-845x hardware support all voltage levels. Please consult your hardware documentation for more information."
        # "Step 2: Create the script and configure the SPI bus:\na) Create the script\nb) Switch the SPI bus pins into master mode. \n    This automatically sets all CS lines to be high.\nc) Configure the Phase and Plarity to mode 0, in \n    which the polarity and phase are both set to \n    zero, however this may be configured for \n    other EEPROMs. \nd) Configure the Clock rate as set by the front \n    panel control."
        # "Your code here.\n(You can make a copy of, or modify, this frame)"
        n72 = Unbundle By Name(w238) -> ("Chip Select"=w232:u32, "Clock Rate (kHz)"=w233:u16, "NI8451 Device ID"=w237:T3, "I/O Voltage Level"=w236:i32, "clock polarity"=w228:i32, "clock phase"=w227:i32, "CS Idle"=w229:enum16{"Low (Assert High)", "High (Assert Low)"})
        n73 = property on="Property Node" class="NI-845x Device"(reference=w237, error in=w231, "IoVoltLevel"=w236) -> (error out=w242:errorcluster)  [unwired: 1 out]
        n74 = call <vilib>:"NI-845x SPI Create Script Reference.vi"("error in (no error)"=w242) -> ("error out"=w241:errorcluster, "spi script reference"=w234:T1)  [unwired: 9 out]
        n75 = call <vilib>:"NI-845x SPI Script Enable SPI.vi"("error in (no error)"=w241, "spi script reference in"=w234) -> ("error out"=w243:errorcluster, "spi script reference out"=w244:T1)  [unwired: 8 out]
        n76 = Bundle By Name(cluster=w238, "SPI Script Reference"=w234) -> (w235:T6)
        n77 = call <vilib>:"NI-845x SPI Script Clock Polarity Phase.vi"("error in (no error)"=w243, "clock phase (0)"=w227, "clock polarity (0)"=w228, "spi script reference in"=w244) -> ("error out"=w239:errorcluster, "spi script reference out"=w240:T1)  [unwired: 2 in, 4 out]
        n78 = call <vilib>:"NI-845x SPI Script Clock Rate.vi"("error in (no error)"=w239, "clock rate in kHz (1000)"=w233, "spi script reference in"=w240) -> ("error out"=w245:errorcluster, "spi script reference out"=w246:T1)  [unwired: 1 in, 6 out]
        n79 = case shown="\"Low (Assert High)\"" w229 {
          tunnel: w246 -> [w252 w256]
          tunnel: w245 -> [w251 w255]
          tunnel: w232 -> [w250 w254]
          tunnel: [w249 w253] -> w230
          frame "Low (Assert High)" {
            # "The Microchip 93C86 CS idle\nstate is LOW and asserted HIGH"
            n80 = call <vilib>:"NI-845x SPI Script CS Low.vi"("error in (no error)"=w251, "chip select (0)"=w250, "spi script reference in"=w252) -> ("error out"=w249:errorcluster)  [unwired: 7 in, 1 out]
          }
          frame "High (Assert Low)" {
            n81 = call <vilib>:"NI-845x SPI Script CS High.vi"("error in (no error)"=w255, "chip select (0)"=w254, "spi script reference in"=w256) -> ("error out"=w253:errorcluster)  [unwired: 7 in, 1 out]
          }
        }
        n82 = call <vilib>:"Add State(s) to Queue__JKI_lib_State_Machine.vi"("State(s) in (\"\")"=w248) -> ("States Out"=w247:string)  [unwired: 14 in]
      }
      frame "NI8451: EWEN" {
        w268 = u8 0
        # "1. Send SB & EWEN Opcode\n2. A dummy address byte\n3. A dummy data byte"
        # "The Microchip 93C86 CS idle\nstate is LOW and asserted HIGH"
        # "EWEN"
        # "Your code here.\n(You can make a copy of, or modify, this frame)"
        n83 = Unbundle By Name(w260) -> ("EWEN"=w257:u8, "SPI Script Reference"=w259:T1, "CS Idle"=w258:enum16{"Low (Assert High)", "High (Assert Low)"})
        n84 = case shown="\"High (Assert Low)\", Default" w258 {
          tunnel: [w280 w284] -> w264
          tunnel: [w279 w283] -> w263
          tunnel: w262 -> [w278 w282]
          tunnel: w259 -> [w277 w281]
          frame "Low (Assert High)" {
            n85 = call <vilib>:"NI-845x SPI Script CS High.vi"("error in (no error)"=w278, "spi script reference in"=w277) -> ("error out"=w279:errorcluster, "spi script reference out"=w280:T1)  [unwired: 8 in]
          }
          frame "High (Assert Low)", Default {
            n86 = call <vilib>:"NI-845x SPI Script CS Low.vi"("error in (no error)"=w282, "spi script reference in"=w281) -> ("error out"=w283:errorcluster, "spi script reference out"=w284:T1)  [unwired: 8 in]
          }
        }
        n87 = Build Array(w257, w268, w268) -> (w267:u8[])
        n88 = call <vilib>:"NI-845x SPI Script Write Read.vi"("error in (no error)"=w263, "write data"=w267, "spi script reference in"=w264) -> ("error out"=w265:errorcluster, "spi script reference out"=w266:T1)  [unwired: 1 in, 6 out]
        n89 = case shown="\"Low (Assert High)\"" w258 {
          tunnel: w266 -> [w273 w276]
          tunnel: w265 -> [w272 w275]
          tunnel: [w271 w274] -> w261
          frame "High (Assert Low)" {
            n90 = call <vilib>:"NI-845x SPI Script CS High.vi"("error in (no error)"=w272, "spi script reference in"=w273) -> ("error out"=w271:errorcluster)  [unwired: 8 in, 1 out]
          }
          frame "Low (Assert High)" {
            n91 = call <vilib>:"NI-845x SPI Script CS Low.vi"("error in (no error)"=w275, "spi script reference in"=w276) -> ("error out"=w274:errorcluster)  [unwired: 8 in, 1 out]
          }
        }
        n92 = call <vilib>:"Add State(s) to Queue__JKI_lib_State_Machine.vi"("State(s) in (\"\")"=w270) -> ("States Out"=w269:string)  [unwired: 14 in]
      }
      frame "NI8451: WRITE" {
        # "Step 3: Generate and write the data to the EEPROM. The format for this EEPROM is:\na) The first byte is 0x5, which is the write opcode. Some EEPROMs require that the 4th bit \nof the opcode be the 9th bit of the EEPROM address,however this is typically only true \nfor single byte addresses.\nb) The next two bytes or byte are the address to write to. Check the correct endianess \nfor your device to sent in big endian format (MSB first) or little endian format (LSB first).\nc) The next x bytes sent to the device are the bytes that are to written to the EEPROM. \nFor this example, we are creating an array of x sequential bytes (0, 1, ...). \nWrites must typically be page-aligned, or else the EEPROM overwrites when it hits a page boundary.\n\nNote: The SubVI calculates the correct EEPROM start addresses for multiple page writes."
        # "Template Separator\n(You can make a copy of, or modify, this frame)"
        n93 = Unbundle By Name(w296) -> ("CS Idle"=w285:enum16{"Low (Assert High)", "High (Assert Low)"}, "Data Address Width"=w290:enum16{"1 Byte", "2 Byte"}, "Page Write Delay (ms)"=w291:u32, "SPI Script Reference"=w295:T1, "Data Address Endianness"=w289:bool, "WRITE"=w286:u8, "EEPROM Data Address"=w294:u8, "Number of Bytes (Read/Write)"=w293:u32, "Target Page Size (bytes)"=w292:u32)
        n94 = case shown="\"All ONES\", Default" "Bit Pattern" {
          tunnel: [255 0 170 85] -> w300
          frame "All ONES", Default {
          }
          frame "All ZEROES" {
          }
          frame "0xAA (0b10101010)" {
          }
          frame "0x55 (0b01010101)" {
          }
        }
        n95 = Quotient & Remainder(x=w293, y=w292) -> (floor(x/y)=w302:u32)  [unwired: 1 out]
        n96 = for {
          N: w293 -> [_]
          tunnel: [w374] -> w301 mode=indexing
          tunnel: w300 -> [w373]
          n97 = To Unsigned Byte Integer(number=w373) -> (unsigned 8bit integer=w374:u8)
        }
        "Data Bytes Written" <- w301
        n98 = for {
          N: w302 -> [_]
          tunnel: w301 -> [w329]
          shift-right: [w328] -> w297
          shift-left: w298 -> [w326]
          shift-right: [w327] -> _
          shift-left: w295 -> [w325]
          tunnel: [w315] -> w287
          tunnel: w302 -> [w311]
          tunnel: w294 -> [w310]
          tunnel: w291 -> [w309]
          tunnel: w290 -> [w308]
          tunnel: w289 -> [w307]
          tunnel: w286 -> [w306]
          tunnel: w285 -> [w305]
          # "The Microchip 93C86 CS idle state is LOW and asserted HIGH"
          # "rotate MSB to low byte\nfor little endian"
          n99 = call-poly <vilib>:"NI-845x SPI Script Delay.vi"("error in (no error)"=w326, "delay in milliseconds (0)"=w309, "spi script reference in"=w325) -> ("error out"=w317:errorcluster, "spi script reference out"=w316:T1)  [unwired: 7 out]
          n100 = Select(t=i16 0, s=w307, f=i16 -8) -> (s? t:f=w320:i16)
          n101 = Rotate(1:w310, 2:w320) -> (0:w313:u8)
          n102 = case shown="\"Low (Assert High)\"" w305 {
            tunnel: [w341 w345] -> w319
            tunnel: [w340 w344] -> w318
            tunnel: w317 -> [w339 w343]
            tunnel: w316 -> [w338 w342]
            frame "High (Assert Low)" {
              n103 = call <vilib>:"NI-845x SPI Script CS Low.vi"("error in (no error)"=w339, "spi script reference in"=w338) -> ("error out"=w340:errorcluster, "spi script reference out"=w341:T1)  [unwired: 8 in]
            }
            frame "Low (Assert High)" {
              n104 = call <vilib>:"NI-845x SPI Script CS High.vi"("error in (no error)"=w343, "spi script reference in"=w342) -> ("error out"=w344:errorcluster, "spi script reference out"=w345:T1)  [unwired: 8 in]
            }
          }
          n105 = Array Subset(array=w329, length=w311) -> (w312:u8[])  [unwired: 1 in]
          n106 = case shown="\"1 Byte\"" w308 {
            tunnel: [w362 w368] -> w314
            tunnel: w313 -> [w361 w364]
            tunnel: w306 -> [w351 w365]
            tunnel: w307 -> [w359 _]
            tunnel: w312 -> [w350 w363]
            tunnel: w310 -> [w346 _]
            frame "1 Byte" {
              n107 = Number To Boolean Array(number=w346) -> (Boolean array=w349:bool[])
              n108 = Number To Boolean Array(number=w351) -> (Boolean array=w356:bool[])
              n109 = Index Array(array=w349, index=8) -> (element=w347:bool)
              n110 = Replace Array Subset(array=w356, new element=w347, index=3) -> (w354:bool[])
              n111 = Split Number(x=w361) -> (hi(x)=w360:u8, lo(x)=w358:u8)
              n112 = Boolean Array To Number(Boolean array=w354) -> (number=w353:u32)
              n113 = To Unsigned Byte Integer(number=w353) -> (unsigned 8bit integer=w352:u8)
              n114 = Select(t=w358, s=w359, f=w360) -> (s? t:f=w357:u8)
              n115 = Build Array (concatenate)(w352, w357, w350) -> (w362:u8[])
            }
            frame "2 Byte", Default {
              # "For MC93C86 the MSB\nis transmitted first\n(high endian)"
              n116 = Split Number(x=w364) -> (hi(x)=w366:u8, lo(x)=w367:u8)
              n117 = Build Array (concatenate)(w365, w366, w367, w363) -> (w368:u8[])
            }
          }
          n118 = call <vilib>:"NI-845x SPI Script Write Read.vi"("error in (no error)"=w318, "write data"=w314, "spi script reference in"=w319) -> ("error out"=w324:errorcluster, "script read index"=w315:u32, "spi script reference out"=w323:T1)  [unwired: 1 in, 5 out]
          n119 = case shown="\"High (Assert Low)\"" w305 {
            tunnel: [w333 w337] -> w328
            tunnel: [w332 w336] -> w327
            tunnel: w324 -> [w331 w335]
            tunnel: w323 -> [w330 w334]
            frame "High (Assert Low)" {
              n120 = call <vilib>:"NI-845x SPI Script CS Low.vi"("error in (no error)"=w331, "spi script reference in"=w330) -> ("error out"=w333:errorcluster, "spi script reference out"=w332:T1)  [unwired: 8 in]
            }
            frame "Low (Assert High)" {
              n121 = call <vilib>:"NI-845x SPI Script CS High.vi"("error in (no error)"=w335, "spi script reference in"=w334) -> ("error out"=w337:errorcluster, "spi script reference out"=w336:T1)  [unwired: 8 in]
            }
          }
        }
        n122 = Bundle By Name(cluster=w296, "script read index"=w287) -> (w288:T6)
        n123 = call <vilib>:"Add State(s) to Queue__JKI_lib_State_Machine.vi"("State(s) in (\"\")"=w304) -> ("States Out"=w303:string)  [unwired: 14 in]
      }
      frame "NI8451: READ" {
        # "Template Separator\n(You can make a copy of, or modify, this frame)"
        n124 = Unbundle By Name(w386) -> ("Chip Select"=w387:u32, "CS Idle"=w377:enum16{"Low (Assert High)", "High (Assert Low)"}, "SPI Script Reference"=w388:T1, "Data Address Width"=w381:enum16{"1 Byte", "2 Byte"}, "READ"=w378:u8, "Data Address Endianness"=w380:bool, "EEPROM Data Address"=w383:u8, "Number of Bytes (Read/Write)"=w382:u32, "Target Page Size (bytes)"=w379:u32)
        n125 = case shown="\"Low (Assert High)\"" w377 {
          tunnel: [w415 w420] -> w398
          tunnel: [w414 w419] -> w397
          tunnel: w388 -> [w413 w418]
          tunnel: w387 -> [w412 w417]
          tunnel: w385 -> [w411 w416]
          frame "High (Assert Low)", Default {
            n126 = call <vilib>:"NI-845x SPI Script CS Low.vi"("error in (no error)"=w411, "chip select (0)"=w412, "spi script reference in"=w413) -> ("error out"=w415:errorcluster, "spi script reference out"=w414:T1)  [unwired: 7 in]
          }
          frame "Low (Assert High)" {
            n127 = call <vilib>:"NI-845x SPI Script CS High.vi"("error in (no error)"=w416, "chip select (0)"=w417, "spi script reference in"=w418) -> ("error out"=w420:errorcluster, "spi script reference out"=w419:T1)  [unwired: 7 in]
          }
        }
        n128 = Select(t=i16 0, s=w380, f=i16 -8) -> (s? t:f=w393:i16)
        n129 = Rotate(1:w383, 2:w393) -> (0:w392:u8)
        n130 = Quotient & Remainder(x=w382, y=w379) -> (floor(x/y)=w390:u32)  [unwired: 1 out]
        n131 = Initialize Array(u32 0 ("element"), w390) -> (w391:u32[])
        n132 = case shown="\"2 Byte\", Default" w381 {
          tunnel: w392 -> [w436 w441]
          tunnel: [w437 w439] -> w396
          tunnel: w378 -> [w431 w440]
          tunnel: w380 -> [w432 _]
          tunnel: w391 -> [w421 w438]
          tunnel: w383 -> [w422 _]
          frame "1 Byte" {
            n133 = Number To Boolean Array(number=w422) -> (Boolean array=w424:bool[])
            n134 = Number To Boolean Array(number=w431) -> (Boolean array=w430:bool[])
            n135 = Index Array(array=w424, index=8) -> (element=w423:bool)
            n136 = Replace Array Subset(array=w430, new element=w423, index=3) -> (w428:bool[])
            n137 = Split Number(x=w436) -> (hi(x)=w434:u8, lo(x)=w435:u8)
            n138 = Boolean Array To Number(Boolean array=w428) -> (number=w427:u32)
            n139 = To Unsigned Byte Integer(number=w427) -> (unsigned 8bit integer=w426:u8)
            n140 = Select(t=w435, s=w432, f=w434) -> (s? t:f=w433:u8)
            n141 = Build Array (concatenate)(w426, w433, w421) -> (w437:u32[])
          }
          frame "2 Byte", Default {
            n142 = Split Number(x=w441) -> (hi(x)=w443:u8, lo(x)=w442:u8)
            n143 = Build Array (concatenate)(w440, w443, w442, w438) -> (w439:u32[])
          }
        }
        n144 = call <vilib>:"NI-845x SPI Script Write Read.vi"("error in (no error)"=w398, "write data"=w396, "spi script reference in"=w397) -> ("error out"=w400:errorcluster, "script read index"=w375:u32, "spi script reference out"=w399:T1)  [unwired: 1 in, 5 out]
        n145 = case shown="\"Low (Assert High)\"" w377 {
          tunnel: w400 -> [w406 w410]
          tunnel: w399 -> [w405 w409]
          tunnel: w387 -> [w404 w408]
          tunnel: [w403 w407] -> w384
          frame "High (Assert Low)", Default {
            n146 = call <vilib>:"NI-845x SPI Script CS High.vi"("error in (no error)"=w406, "chip select (0)"=w404, "spi script reference in"=w405) -> ("error out"=w403:errorcluster)  [unwired: 7 in, 1 out]
          }
          frame "Low (Assert High)" {
            n147 = call <vilib>:"NI-845x SPI Script CS Low.vi"("error in (no error)"=w410, "chip select (0)"=w408, "spi script reference in"=w409) -> ("error out"=w407:errorcluster)  [unwired: 7 in, 1 out]
          }
        }
        n148 = Bundle By Name(cluster=w386, "script read index"=w375) -> (w376:T6)
        n149 = call <vilib>:"Add State(s) to Queue__JKI_lib_State_Machine.vi"("State(s) in (\"\")"=w402) -> ("States Out"=w401:string)  [unwired: 14 in]
      }
      frame "NI8451: EWDS" {
        w454 = u8 0
        # "1. Send SB & EWDS Opcode\n2. A dummy address byte\n3. A dummy data byte"
        # "Step 4: Finish and run the script\na) send the EWDS (Write Disable) instruction\na) Disable the SPI bus by configuring the SPI \n    interface pins to hi-z.\nb) Run the script on the passed-in device. \nc) Close the script reference to delete the \n    script."
        # "Template Separator\n(You can make a copy of, or modify, this frame)"
        n150 = Unbundle By Name(w448) -> ("EWDS"=w444:u8, "SPI Script Reference"=w446:T1, "Chip Select"=w447:u32)
        n151 = call <vilib>:"NI-845x SPI Script CS High.vi"("error in (no error)"=w450, "chip select (0)"=w447, "spi script reference in"=w446) -> ("spi script reference out"=w445:T1)  [unwired: 7 in, 1 out]
        n152 = Build Array(w444, w454, w454) -> (w453:u8[])
        n153 = call <vilib>:"NI-845x SPI Script Write Read.vi"("error in (no error)"=w450, "write data"=w453, "spi script reference in"=w445) -> ("error out"=w451:errorcluster, "spi script reference out"=w452:T1)  [unwired: 1 in, 6 out]
        n154 = call <vilib>:"NI-845x SPI Script CS Low.vi"("error in (no error)"=w451, "spi script reference in"=w452) -> ("error out"=w449:errorcluster)  [unwired: 8 in, 1 out]
        n155 = call <vilib>:"Add State(s) to Queue__JKI_lib_State_Machine.vi"("State(s) in (\"\")"=w456) -> ("States Out"=w455:string)  [unwired: 14 in]
      }
      frame "NI8451: Close SPI and RUN Script" {
        # "Template Separator\n(You can make a copy of, or modify, this frame)"
        n156 = Unbundle By Name(w467) -> ("Data Address Width"=w459:enum16{"1 Byte", "2 Byte"}, "script read index"=w460:u32, "NI8451 Device ID"=w457:T3, "SPI Script Reference"=w468:T1)
        n157 = call <vilib>:"NI-845x SPI Script Disable SPI.vi"("error in (no error)"=w470, "spi script reference in"=w468) -> ("error out"=w471:errorcluster, "spi script reference out"=w472:T1)  [unwired: 8 out]
        n158 = case shown="\"1 Byte\"" w459 {
          tunnel: [2 ("index") 3 ("index")] -> w458
          frame "1 Byte" {
          }
          frame "2 Byte", Default {
          }
        }
        n159 = call <vilib>:"NI-845x SPI Run Script.vi"("error in (no error)"=w471, "device reference in"=w457, "spi script reference in"=w472) -> ("error out"=w464:errorcluster, "spi script reference out"=w465:T1)  [unwired: 1 in, 6 out]
        n160 = call <vilib>:"NI-845x SPI Extract Script Read Data.vi"("error in (no error)"=w464, "script read index"=w460, "spi script reference in"=w465) -> ("error out"=w463:errorcluster, "read data"=w461:u8[], "spi script reference out"=w462:T1)  [unwired: 6 out]
        n161 = Array Subset(array=w461, index=w458) -> (→"Read Data":u8[])  [unwired: 1 in]
        n162 = call-poly <vilib>:"NI-845x Close Reference.vi"("error in (no error)"=w463, "spi script reference"=w462) -> ("error out"=w469:errorcluster)  [unwired: 9 out]
        n163 = call <vilib>:"Add State(s) to Queue__JKI_lib_State_Machine.vi"("State(s) in (\"\")"=w474) -> ("States Out"=w473:string)  [unwired: 14 in]
      }
    }
  }
